vi "Get Analog Input Type.vi"(8 "error in (no error)":errorcluster, 11 "VISA resource name":refnum<visa-resource-name>) -> (0 "error out":errorcluster, 1 "Analog Input Type (out)":enum16{"Voltage", "Current"}(ring), 3 "VISA resource name out":refnum<visa-resource-name>)   [LabVIEW 2015, in "JULABO DeviceDriver.lvlib"]
doc: "This VI returns the type of external programmer input:\n0 = Voltage 0 V to 10 V\n1 = Current 0 mA to 20 mA\n\nNote:\nThis function is not available for all instruments. See operating manual to check whether your instrument supports this feature."
uses:
  JULABO DeviceDriver.lvlib
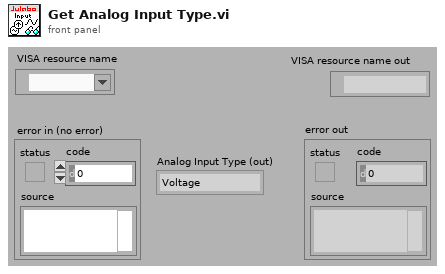
[diagram p1: front panel]
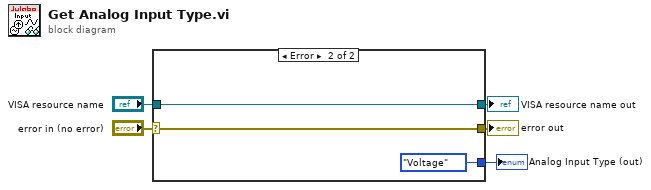
[diagram p0: block diagram]
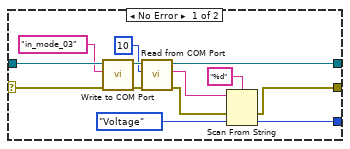
[diagram p2: hidden frame]
diagram:
  n1 = case shown="Error" "error in (no error)" {
    selector: "error in (no error)" -> [w17 w20]
    tunnel: "VISA resource name" -> [w18 w21]
    tunnel: [w11 w20] -> w3
    tunnel: [w10 w21] -> w2
    tunnel: [w7 enum16{"Voltage", "Current"}."Voltage" ("Analog Input Type (out)")] -> w1
    frame No Error {
      n2 = call "Write to COM Port.vi"("error in"=w17, "Command (input)"="in_mode_03", "VISA resource name in"=w18) -> ("error out"=w16:errorcluster, "VISA resource name out"=w15:refnum<visa-resource-name>)  [unwired: 7 in]
      n3 = call "Read from COM Port.vi"("error in"=w16, "Byte to Read (-1:All)"=u32 10 ("Anzahl der Byte"), "VISA resource name in"=w15) -> ("error out"=w13:errorcluster, "String (output)"=w12:string, "VISA resource name out"=w10:refnum<visa-resource-name>)  [unwired: 5 in, 1 out]
      n4 = Scan From String(format string="%d" ("Format-String"), input string=w12, error in=w13, default 1=enum16{"Voltage", "Current"}."Voltage" ("Analog Input Type (out)")) -> (error out=w11:errorcluster, output 1=w7:enum16{"Voltage", "Current"})  [unwired: 1 in, 2 out]
    }
    frame Error {
    }
  }
  "error out" <- w3
  "VISA resource name out" <- w2
  "Analog Input Type (out)" <- w1
